vi "Check Read Volt.vi"(8 "error in (no error)":errorcluster, 11 "RT Data in in":T1 {"Channels"."Voltage"."Ref"."Data Reference" format="%.0x"; "Channels"."Current"."Ref"."Data Reference" format="%.0x"; "Channels"."Read Volt"."Ref" format="%.0x"; "Channels"."Mode"."Ref" format="%.0x"}) -> (0 "error out":errorcluster, 3 "RT Data out":T1 {"Channels"."Voltage"."Ref"."Data Reference" format="%.0x"; "Channels"."Current"."Ref"."Data Reference" format="%.0x"; "Channels"."Read Volt"."Ref" format="%.0x"; "Channels"."Mode"."Ref" format="%.0x"})   [LabVIEW 2011, in "Switch-DMM Custom Device.lvlib"]
uses:
  Switch-DMM Custom Device.lvlib
  Controls/RT Data.ctl
  Controls/Channels.ctl
  Controls/Single Channel.ctl
  <vilib>/NI Veristand/Custom Device API/Data Reference.ctl
  Controls/Block Channels.ctl
  <vilib>/NI Veristand/Custom Device API/Block Data Reference.ctl
  Controls/Communication.ctl
  Controls/Async Status.ctl
  Controls/Async State.ctl
  Controls/Async Command.ctl
  Controls/Async Events.ctl
  <vilib>/NI Veristand/Custom Device API/Global Data Refs.vi
  <vilib>/NI Veristand/Custom Device API/Custom Device API.lvlib
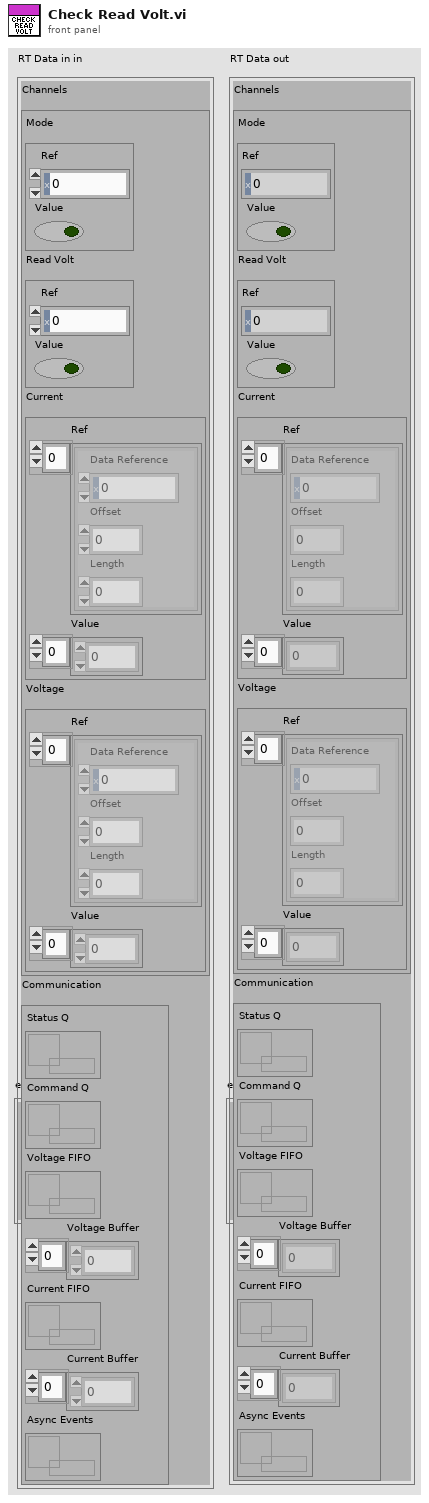
[diagram p1: front panel]
types:
  T1 = typedef "Switch-DMM Custom Device.lvlib/RT Data.ctl" = cluster{"Channels":T2, "Communication":T7}
  T2 = typedef "Switch-DMM Custom Device.lvlib/Channels.ctl" = cluster{"Mode":T3, "Read Volt":T3, "Current":T5, "Voltage":T5}
  T3 = typedef "Switch-DMM Custom Device.lvlib/Single Channel.ctl" = cluster{"Ref":T4, "Value":bool}
  T4 = typedef "Custom Device API.lvlib/Data Reference.ctl" = i32
  T5 = typedef "Switch-DMM Custom Device.lvlib/Block Channels.ctl" = cluster{"Ref":T6[], "Value":dbl[]}
  T6 = typedef "Custom Device API.lvlib/Block Data Reference.ctl" = cluster{"Data Reference":T4, "Offset":i32, "Length":i32}
  T7 = typedef "Switch-DMM Custom Device.lvlib/Communication.ctl" = cluster{"Status Q":refnum<queue>, "Command Q":refnum<queue>, "Voltage FIFO":refnum<k33>, "Voltage Buffer":dbl[], "Current FIFO":refnum<k33>, "Current Buffer":dbl[], "Async Events":refnum<queue>}
  T8 = typedef "Switch-DMM Custom Device.lvlib/Async Command.ctl" = enum16{"None", "Start", "Set Cur Mode", "Req Volt Mode", "Set Volt Mode", "Read Volt", "Exit"}
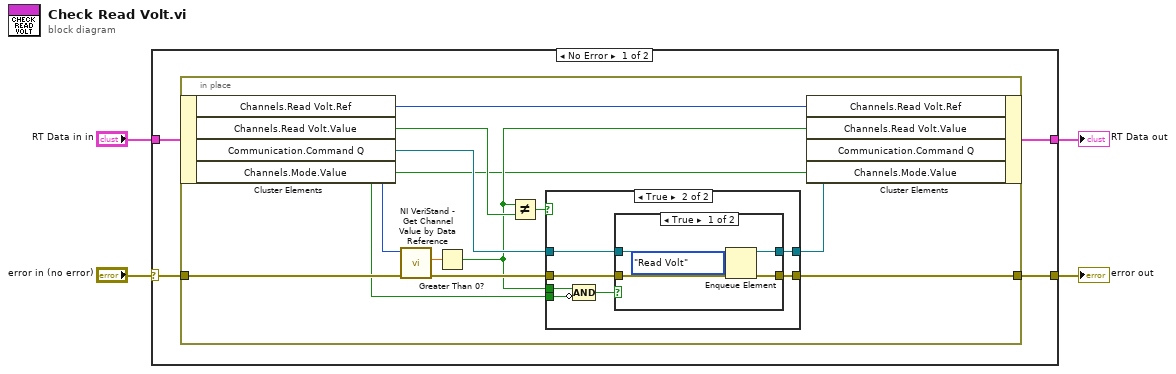
[diagram p0: block diagram]
diagram:
  n1 = case shown="No Error" "error in (no error)" {
    selector: "error in (no error)" -> [w8 w36]
    tunnel: "RT Data in in" -> [w7 w37]
    tunnel: [w6 w37] -> w3
    tunnel: [w5 w36] -> w4
    frame No Error {
      n2 = in-place {
        in-place-border: w8 -> [w18]
        in-place-border: [w11] -> w5
        n3 = in-place-cluster #1(w7) -> ("Channels.Read Volt.Ref"=w19:T4, "Channels.Read Volt.Value"=w17:bool, "Communication.Command Q"=w14:refnum<queue>, "Channels.Mode.Value"=w9:bool)
        n4 = call <vilib>:"NI VeriStand - Get Channel Value by Data Reference.vi"("error in (no error)"=w18, "Data Reference in"=w19) -> ("error out"=w12:errorcluster, "Value"=w15:dbl)  [unwired: 8 in]
        n5 = Greater Than 0?(x=w15) -> (x > 0?=w10:bool)
        n6 = Not Equal?(x=w10, y=w17) -> (x != y?=w16:bool)
        n7 = case shown="True" w16 {
          tunnel: w14 -> [w21 w28]
          tunnel: w10 -> [_ w23]
          tunnel: [w21 w27] -> w13
          tunnel: w12 -> [w20 w26]
          tunnel: [w20 w25] -> w11
          tunnel: w9 -> [_ w22]
          frame False {
          }
          frame True {
            n8 = Compound Arithmetic op=AND(w23, invert w22) -> (w24:bool)
            n9 = case shown="True" w24 {
              tunnel: w28 -> [w33 w35]
              tunnel: [w32 w35] -> w27
              tunnel: w26 -> [w31 w34]
              tunnel: [w29 w34] -> w25
              frame True {
                n10 = Enqueue Element(queue=w33, element=Async_Command."Read Volt", error in (no error)=w31) -> (queue out=w32:refnum<queue>, error out=w29:errorcluster)  [unwired: 1 in, 1 out]
              }
              frame False {
              }
            }
          }
        }
        n11 = in-place-cluster #1("Channels.Read Volt.Ref"=w19, "Channels.Read Volt.Value"=w10, "Communication.Command Q"=w13, "Channels.Mode.Value"=w9) -> (w6:T1)
      }
    }
    frame Error {
    }
  }
  "error out" <- w4
  "RT Data out" <- w3
